vi "output_pid.vi"(7 "dt (s)":dbl=-1.0 format="%.3f", 8 "PID gains":T1, 9 "Input Pulse Per Sec":dbl, 10 "Last Position":i32, 11 "Current Position":i32) -> (1 "Current Speed":i32, 2 "DIR":bool, 3 "PWM Signal":dbl)   [LabVIEW 2016]
uses:
  <vilib>/addons/control/pid/pid.llb/PID (DBL).vi
  <vilib>/addons/control/pid/NI_PID_pid.lvlib
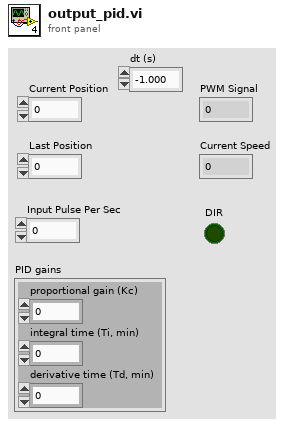
[diagram p1: front panel]
types:
  T1 = cluster{"proportional gain (Kc)":dbl, "integral time (Ti, min)":dbl, "derivative time (Td, min)":dbl}
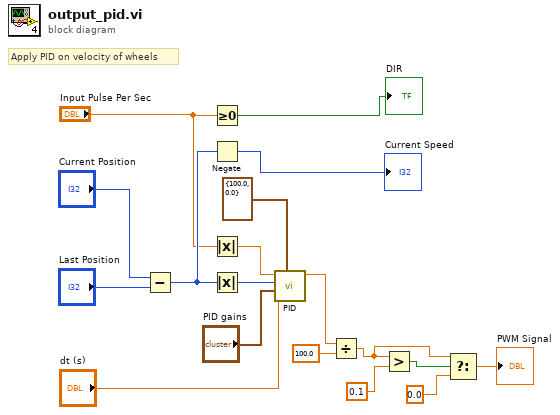
[diagram p0: block diagram]
diagram:
  # "Apply PID on velocity of wheels"
  n1 = Subtract(x="Current Position", y="Last Position") -> (x-y=w17:i32)
  n2 = Greater Or Equal To 0?(x="Input Pulse Per Sec") -> (x >= 0?=→"DIR":bool)
  n3 = Negate(x=w17) -> (-x=→"Current Speed":i32)
  n4 = Absolute Value(x="Input Pulse Per Sec") -> (abs(x)=w14:dbl)
  n5 = Absolute Value(x=w17) -> (abs(x)=w15:i32)
  n6 = call-poly <vilib>:"PID.vi"("output range"=cluster{"output high":dbl, "output low":dbl} {"output high"=100.0, "output low"=0.0}, "dt (s)"="dt (s)", "PID gains"="PID gains", "process variable"=w15, "setpoint"=w14) -> ("output"=w9:dbl)  [unwired: 5 in, 1 out]
  n7 = Divide(x=w9, y=100.0) -> (x/y=w2:dbl)
  n8 = Greater?(x=w2, y=0.1) -> (0:w3:bool)
  n9 = Select(t=w2, s=w3, f=0.0) -> (s? t:f=→"PWM Signal":dbl)
